vi "Other Output Item.vi"(8 "error in (no error)":errorcluster, 9 "Project In":refnum<class "Project.lvclass">, 11 "Output":T1) -> (0 "error out":errorcluster)   [LabVIEW 2015, in "OutputUI.lvclass"]
uses:
  OutputUI.lvclass
  Step/STEP_OUTPUT.ctl
  Step/OUTPUT_DATA_TYPE.ctl
  OUTPUT_CHECK_TYPE.ctl
  Step/OUTPUT_VALUE_TYPE.ctl
  Project.lvclass
  SerializableObject/CONFIGURE_UI_STATE.ctl
  Editor/Editor.lvclass
  Step.lvclass
panel:
  in  "Variable Name":string(combo) caption="Variable Name 1"
  in  "Check":u16(ring)
  out "Type Image":picture
  in  "Output":string
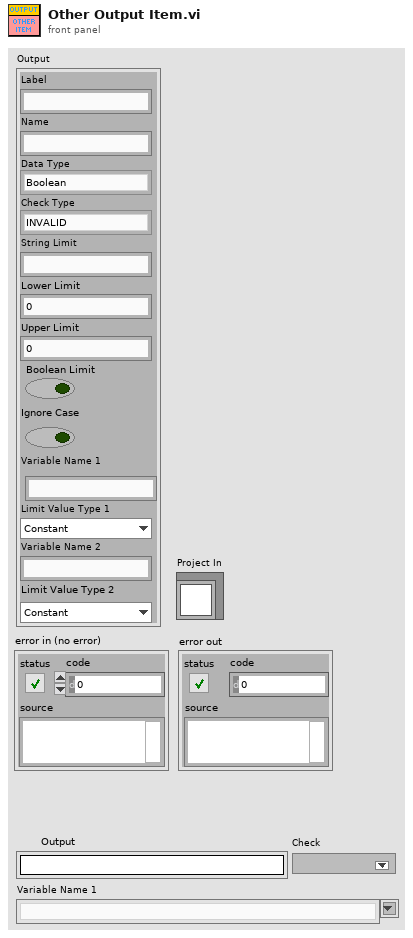
[diagram p1: front panel]
types:
  T1 = typedef "Step.lvclass/STEP_OUTPUT.ctl" = cluster{"Label":string, "Name":string, "Data Type":T2, "Check Type":T3, "String Limit":string, "Lower Limit":dbl, "Upper Limit":dbl, "Boolean Limit":bool, "Ignore Case":bool, "Variable Name 1":string, "Limit Value Type 1":T4, "Variable Name 2":string, "Limit Value Type 2":T4}
  T2 = typedef "Step.lvclass/OUTPUT_DATA_TYPE.ctl" = enum16{"Boolean", "String", "Numeric", "Other"}
  T3 = typedef "Step.lvclass/OUTPUT_CHECK_TYPE.ctl" = enum16{"INVALID", "DO_NOT_CHECK", "RECORD", "VARIABLE", "EQUAL", "NOT_EQUAL", "STR_CONTAINS", "STR_START_WITH", "STR_END_WITH", "STR_REGEX_MATCH", "NUM_GT", "NUM_LT", "NUM_GE", "NUM_LE", "NUM_RANGE", "NUM_RANGE_BDY"}
  T4 = typedef "Step.lvclass/OUTPUT_VALUE_TYPE.ctl" = enum16{"Constant", "Variable"}
  T5 = cluster{"Type Image":refnum<vi>, "Output":refnum<vi>, "Check":refnum<vi>, "Variable Name":refnum<vi>}
  T6 = typedef "Editor.lvclass/CONFIGURE_UI_STATE.ctl" = enum16{"UI_LOOP", "INIT", "END", "CHANGE_PANEL"}
  T7 = typedef "LVRectTypeDef.ctl" = cluster{"Left":i16, "Top":i16, "Right":i16, "Bottom":i16}
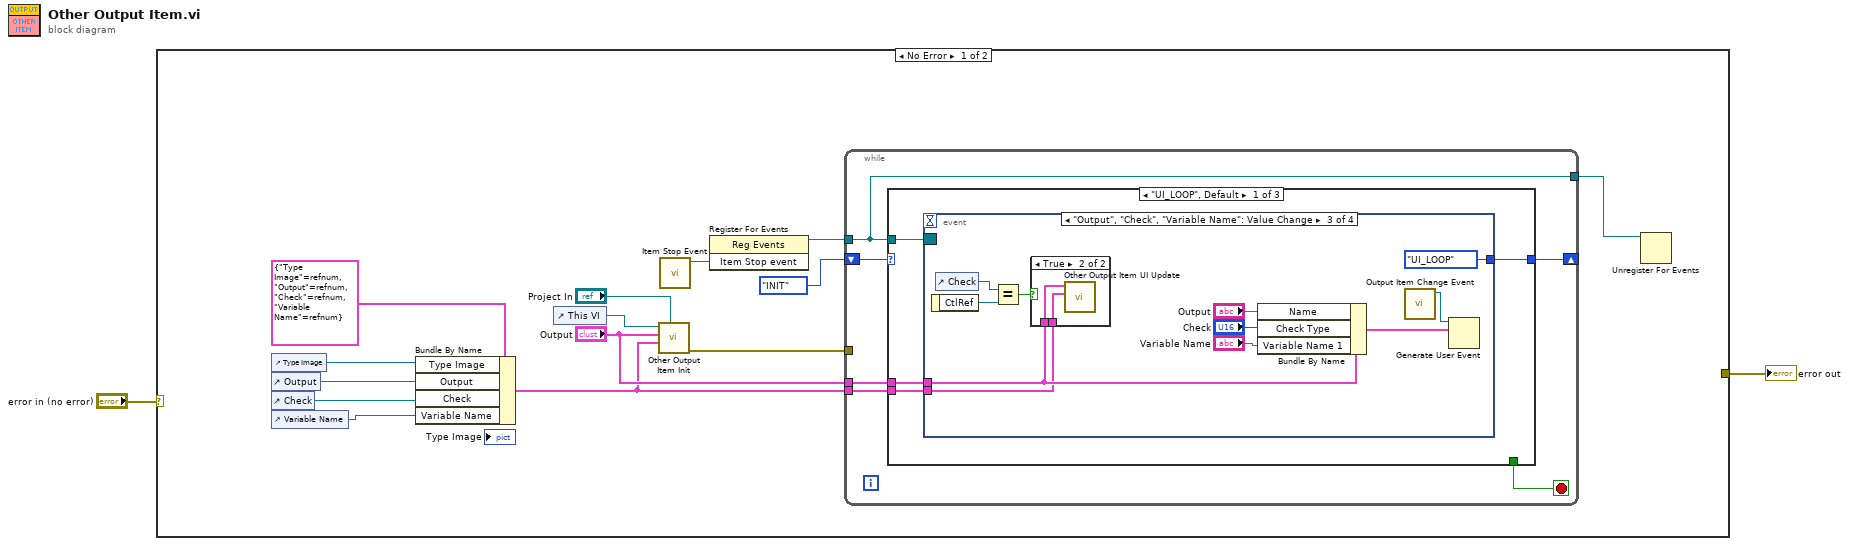
[diagram p0: block diagram]
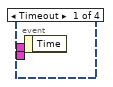
[diagram p2: hidden frame]
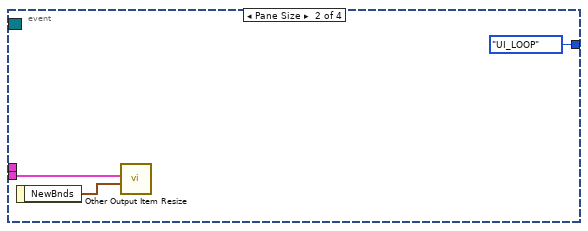
[diagram p3: hidden frame]
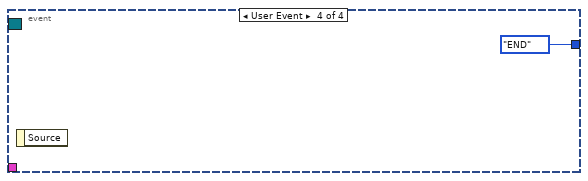
[diagram p5: hidden frame]
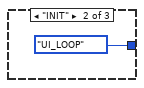
[diagram p6: hidden frame]
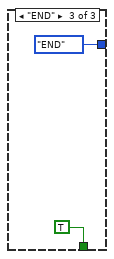
[diagram p7: hidden frame]
diagram:
  n1 = case shown="No Error" "error in (no error)" {
    selector: "error in (no error)" -> [_ w47]
    tunnel: [_ w47] -> w1
    frame No Error {
      n2 = control-ref of="Type Image"() -> (w9:refnum<vi>)
      n3 = control-ref of="Output"() -> (w6:refnum<vi>)
      n4 = control-ref of="Check"() -> (w7:refnum<vi>)
      n5 = control-ref of="Variable Name"() -> (w4:refnum<vi>)
      n6 = Bundle By Name(cluster=T5 {"Type Image"=refnum, "Output"=refnum, "Check"=refnum, "Variable Name"=refnum} ("UI Elements"), "Type Image"=w9, "Output"=w6, "Check"=w7, "Variable Name"=w4) -> (w3:T5)
      n7 = control-ref of="This VI"() -> (w12:refnum<vi>)
      n8 = call "Other Output Item Init.vi"("Project In"="Project In", "Other UI Elements"=w3, "Output"="Output", "VI in"=w12) -> ("error out"=w11:errorcluster)  [unwired: 7 in]
      n9 = call "Item Stop Event.vi"() -> ("Item Stop event"=w15:refnum<user-event>)  [unwired: 11 in]
      n10 = register-events(w15) -> (reference out=w14:refnum<event-registration>)  [unwired: 2 in, 1 out]
      n11 = while {
        shift-right: [w21] -> _
        shift-left: CONFIGURE_UI_STATE."INIT" -> [w22]
        tunnel: w14 -> [w19]
        tunnel: [w19] -> w13
        tunnel: w11 -> [_]
        tunnel: "Output" -> [w18]
        tunnel: w3 -> [w17]
        stop <- w20 stop-if-true
        n12 = case shown="\"UI_LOOP\", Default" w22 {
          tunnel: [w26 CONFIGURE_UI_STATE."UI_LOOP" CONFIGURE_UI_STATE."END"] -> w21
          tunnel: [_ _ TRUE] -> w20
          tunnel: w19 -> [w25 _ _]
          tunnel: w18 -> [w24 _ _]
          tunnel: w17 -> [w23 _ _]
          frame "UI_LOOP", Default {
            n13 = event shown="[2] \"Output\", \"Check\", \"Variable Name\": Value Change" {
              selector: w25 -> [_ _ _ _]
              dyn-events: _ -> [_ _ _ _]
              timeout: _ -> [_ _ _ _]
              tunnel: [_ CONFIGURE_UI_STATE."UI_LOOP" CONFIGURE_UI_STATE."UI_LOOP" CONFIGURE_UI_STATE."END"] -> w26
              tunnel: w24 -> [_ _ w34 _]
              tunnel: w23 -> [_ w29 w33 _]
              event Timeout {
                n14 = event-data() -> ()  [unwired: 1 in, 1 out]
              }
              event Pane Size {
                n15 = event-data() -> ("NewBnds"=w28:T7)  [unwired: 1 in]
                n16 = call "Other Output Item Resize.vi"("NewBnds"=w28, "Other UI Elements"=w29) -> ()  [unwired: 9 in, 1 out]
              }
              event "Output", "Check", "Variable Name": Value Change {
                n17 = event-data() -> ("CtlRef"=w32:refnum<vi>)  [unwired: 1 in]
                n18 = control-ref of="Check"() -> (w35:refnum<vi>)
                n19 = Equal?(x=w35, y=w32) -> (x = y?=w30:bool)
                n20 = case shown="True" w30 {
                  tunnel: w34 -> [_ w42]
                  tunnel: w33 -> [_ w41]
                  frame False {
                  }
                  frame True {
                    n21 = call "Other Output Item UI Update.vi"("Other UI Elements"=w41, "Output"=w42) -> ()  [unwired: 9 in, 1 out]
                  }
                }
                n22 = Bundle By Name(cluster=w34, "Name"="Output", "Check Type"="Check", "Variable Name 1"="Variable Name") -> (w36:T1)
                n23 = call "Output Item Change Event.vi"() -> ("Output Value Change Event"=w37:refnum<user-event>)  [unwired: 11 in]
                n24 = Generate User Event(user event=w37, event data cluster=w36) -> ()  [unwired: 2 in, 2 out]
              }
              event User Event {
                n25 = event-data() -> ()  [unwired: 1 in, 1 out]
              }
            }
          }
          frame "INIT" {
          }
          frame "END" {
          }
        }
      }
      n26 = Unregister For Events(event registration refnum=w13) -> ()  [unwired: 1 in, 1 out]
    }
    frame Error {
    }
  }
  "error out" <- w1
